vi "CharEditor.vi"() -> ()   [LabVIEW 2018]
uses:
  TypDefs/Char_Enum.ctl
panel:
  in  "ReplaceColor":bool
  in  "Color 2":u8(ring)=2
  in  "Color 1":u8(ring)
  out "Blue_LUT":bool[](array[boolean])
  out "Green_LUT":bool[](array[boolean])
  out "Red_LUT":bool[](array[boolean])
  in  "Create LUT":bool
  in  "Fill Column":bool
  in  "Color":u8(ring)
  in  "Fill Row":bool
  in  "Column":i32 min=0 max=24 step=1
  in  "Row":i32 min=0 max=24 step=1
  in  "Clear tile":bool
  in  "Rotate tile":bool
  in  "Paste tile":bool
  in  "Copy tile":bool
  in  "Save Tileset":bool
  in  "Active char":T1
  in  "25x25 Tile":u8[][](array[ring])
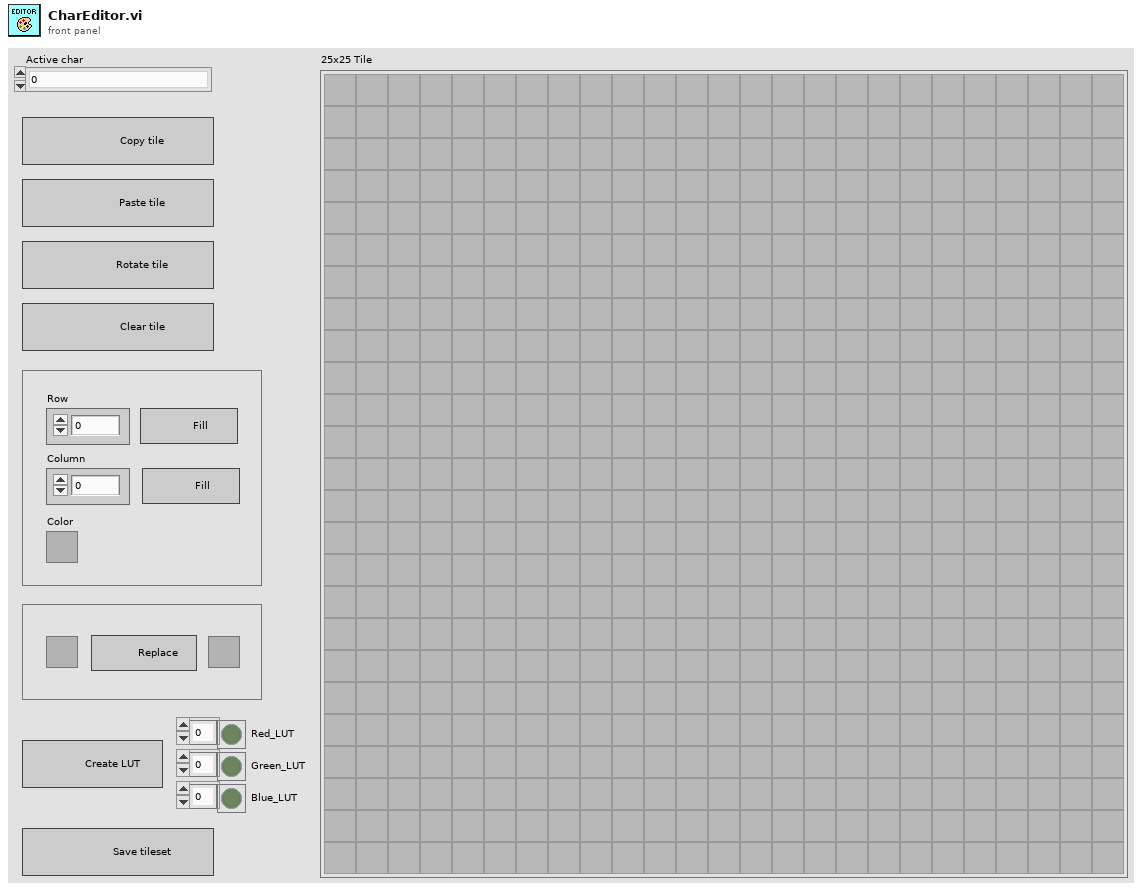
[diagram p1: front panel]
types:
  T1 = typedef "Char_Enum.ctl" = enum8{"0", "1", "2", "3", "4", "5", "6", "7", "8", "9"}
  T2 = cluster{"FilePath":path, "ActiveChar":T1, "TileSizeX":i32, "TileSizeY":i32, "Tileset":u8[][][], "Copy":u8[][]}
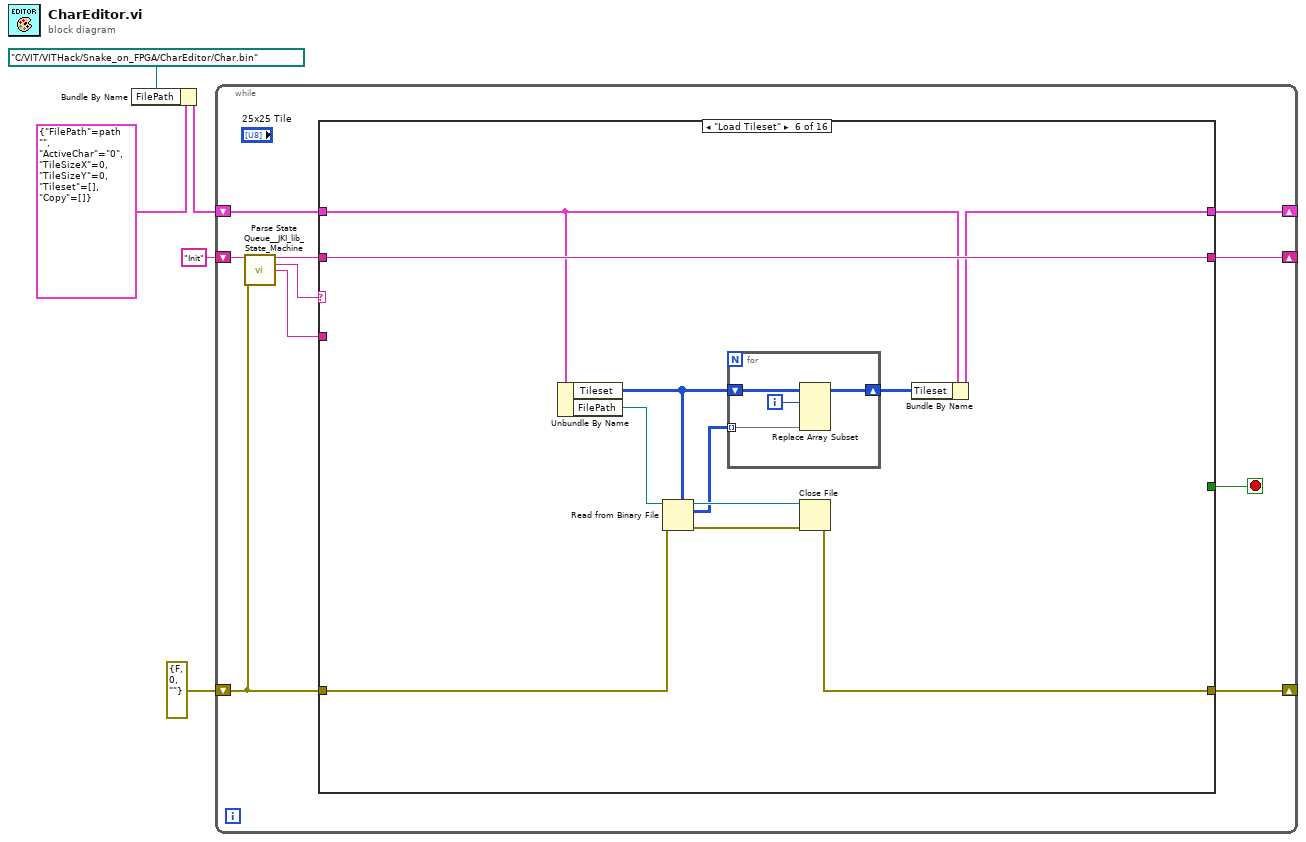
[diagram p0: block diagram]
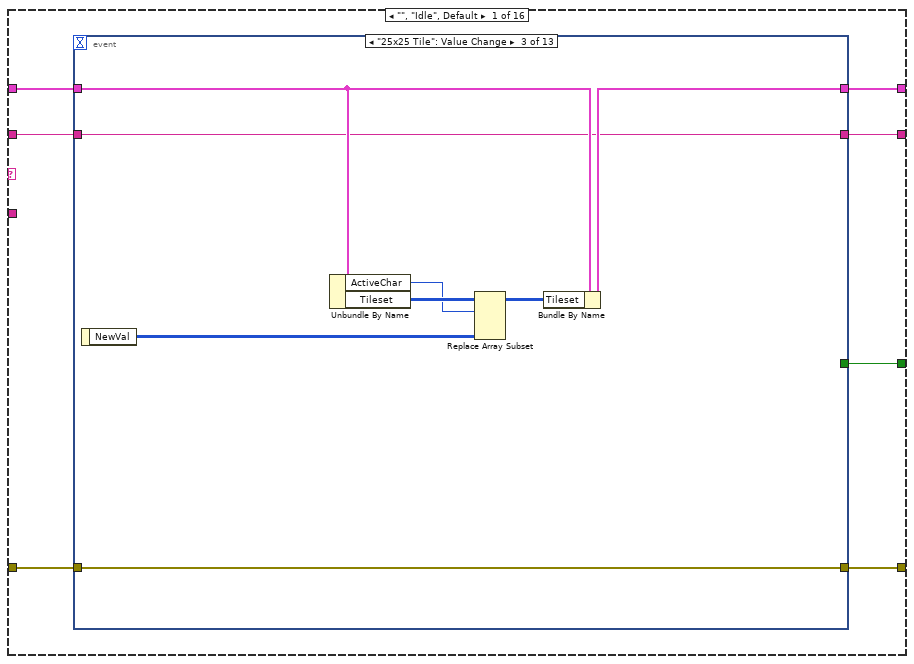
[diagram p2: hidden frame]
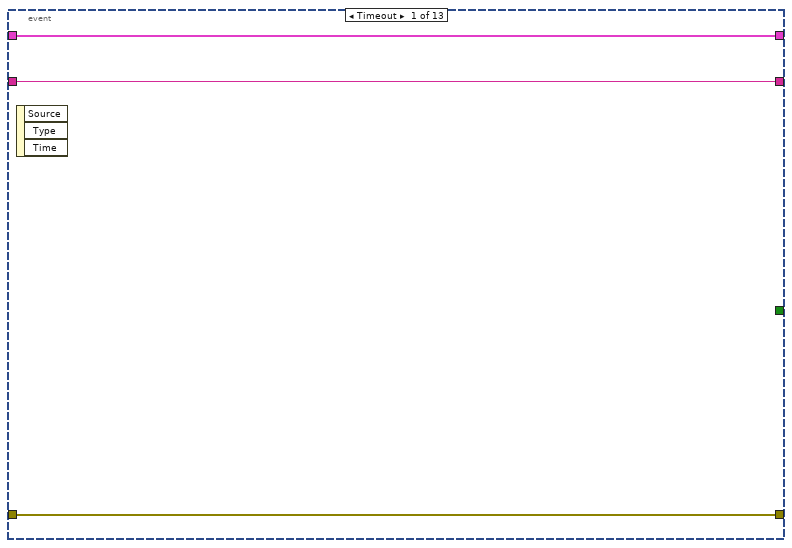
[diagram p3: hidden frame]
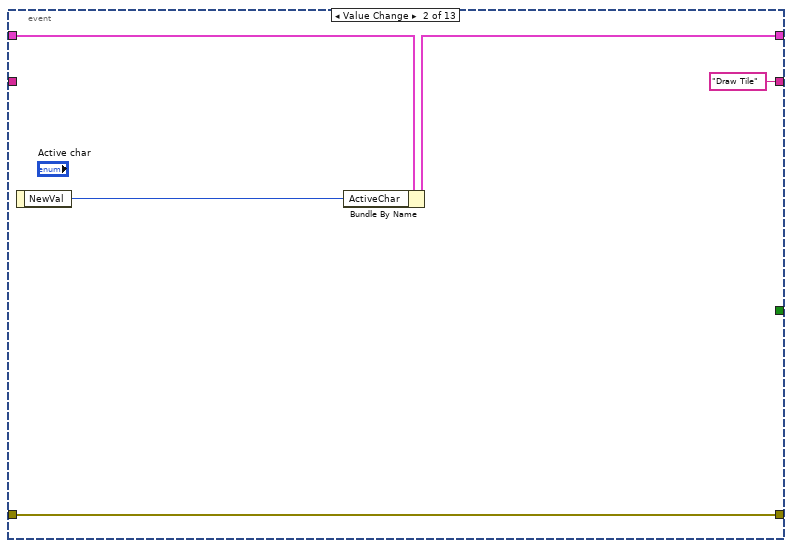
[diagram p4: hidden frame]
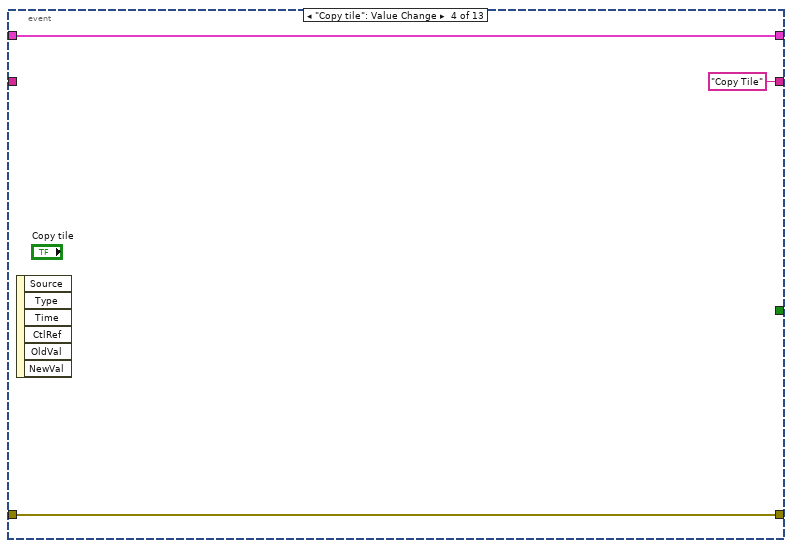
[diagram p5: hidden frame]
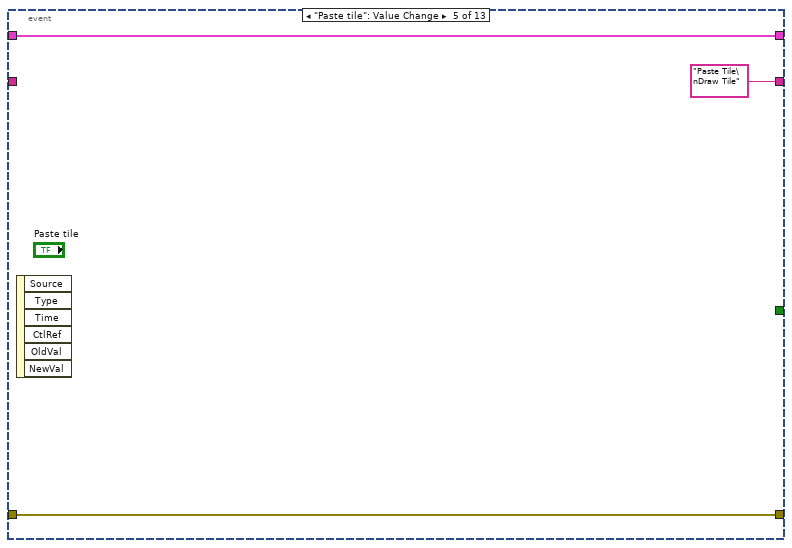
[diagram p6: hidden frame]
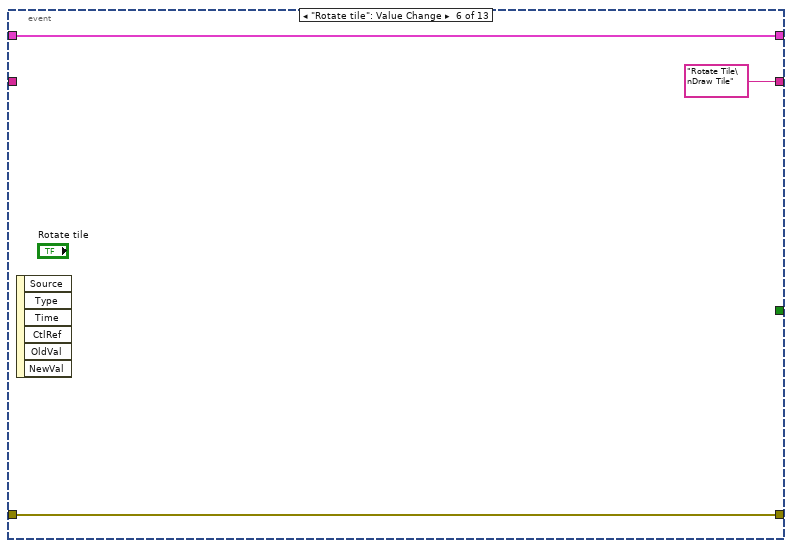
[diagram p7: hidden frame]
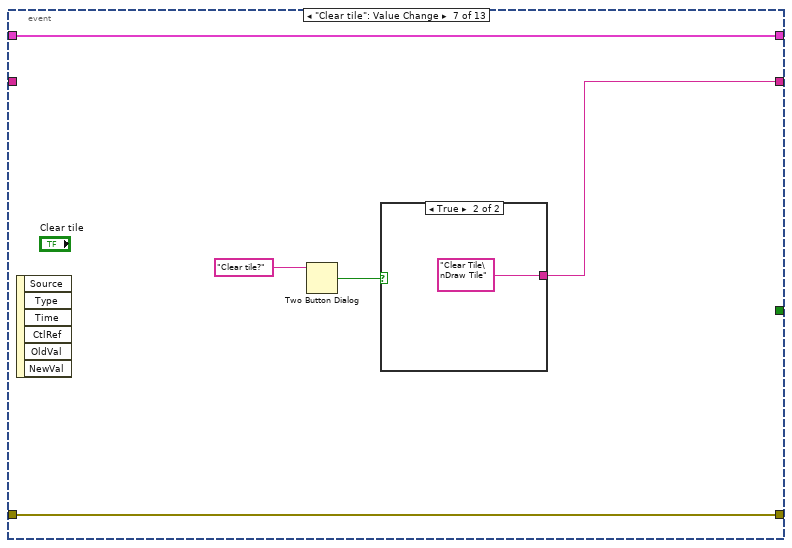
[diagram p8: hidden frame]
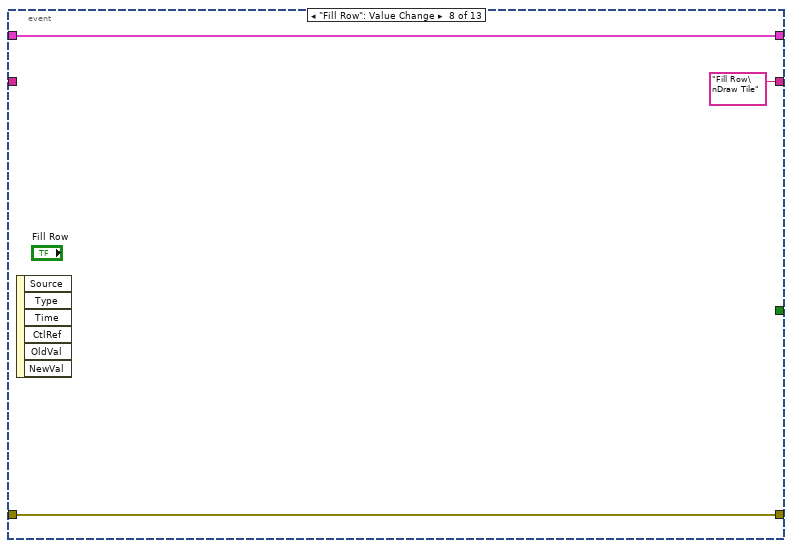
[diagram p10: hidden frame]
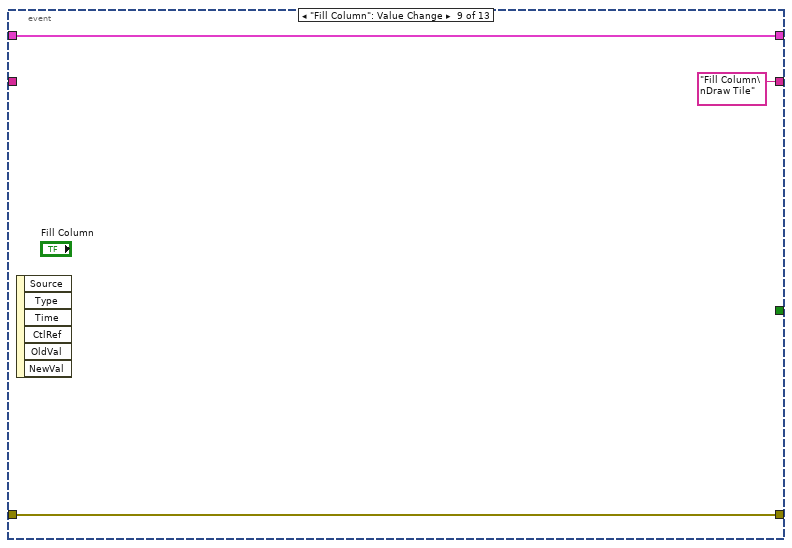
[diagram p11: hidden frame]
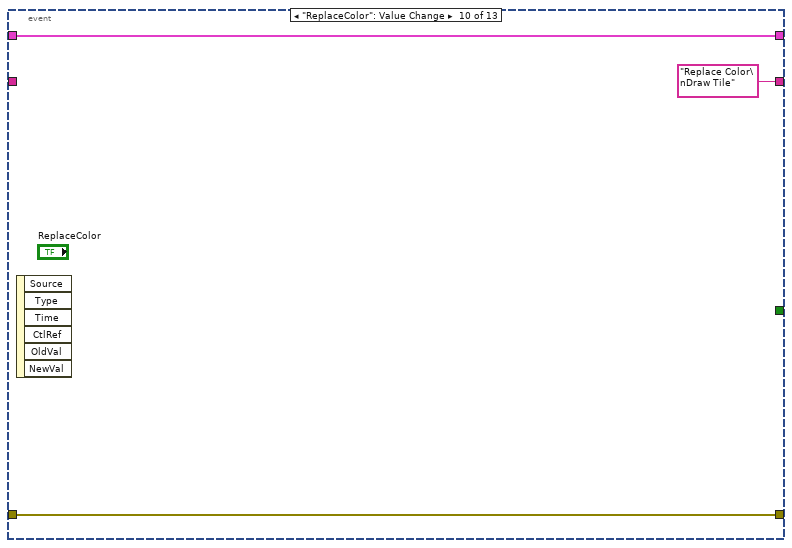
[diagram p12: hidden frame]
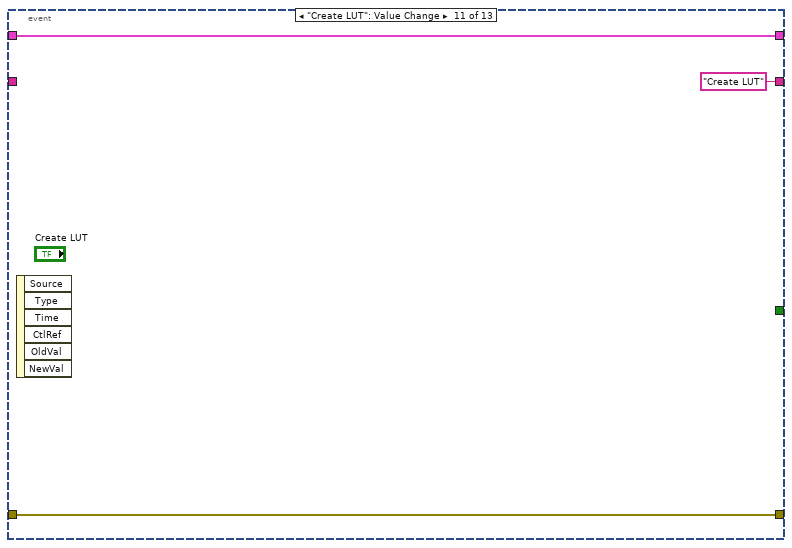
[diagram p13: hidden frame]
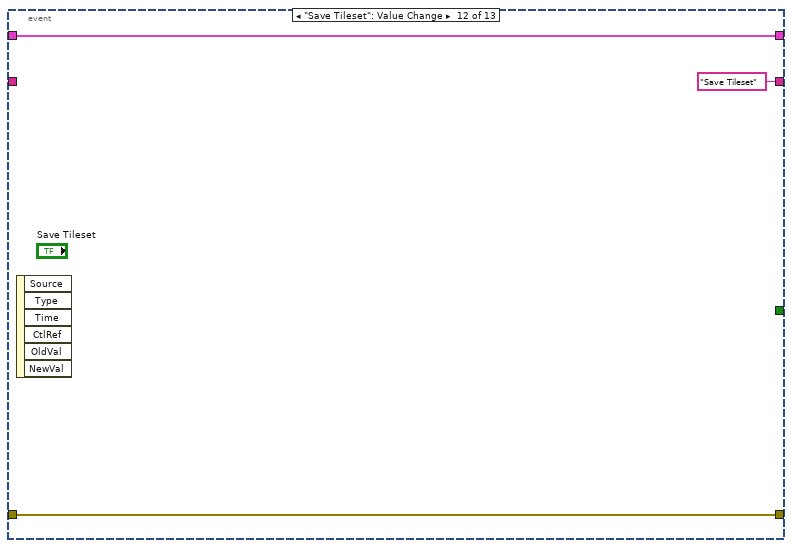
[diagram p14: hidden frame]
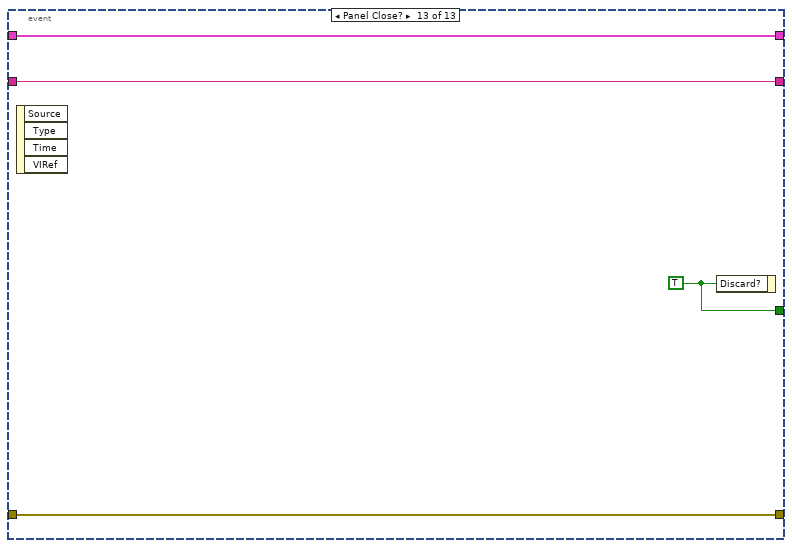
[diagram p15: hidden frame]
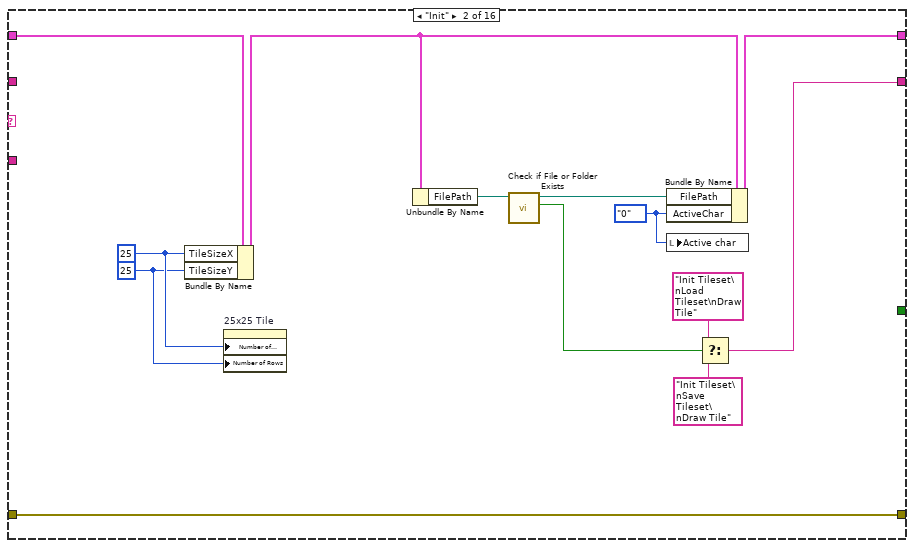
[diagram p16: hidden frame]
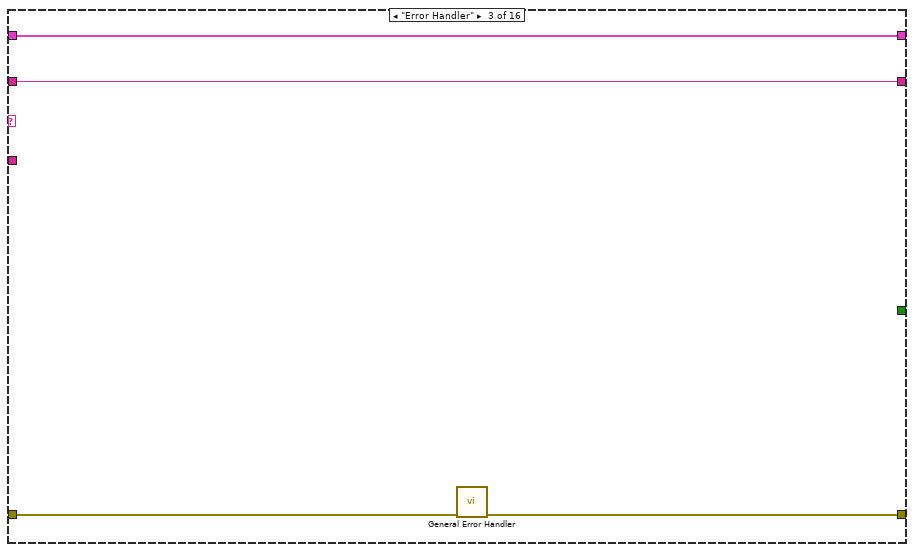
[diagram p17: hidden frame]
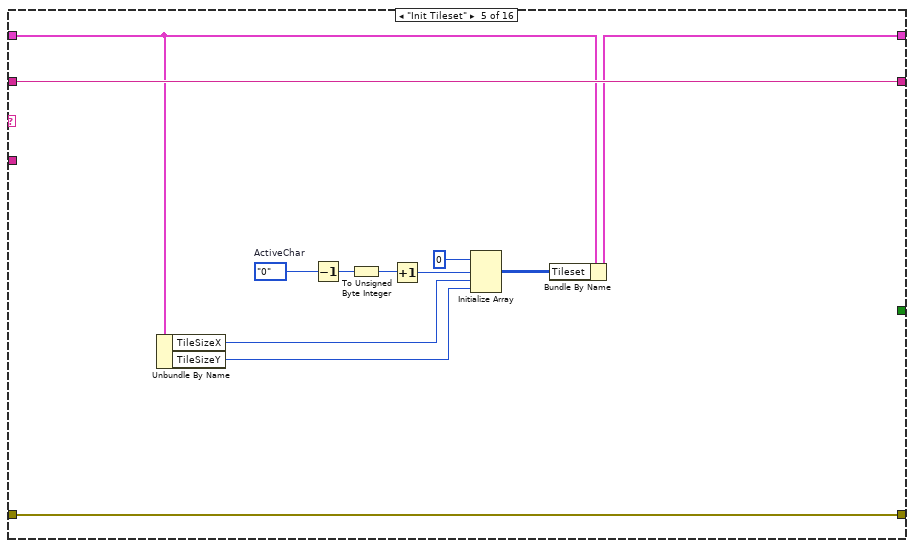
[diagram p19: hidden frame]
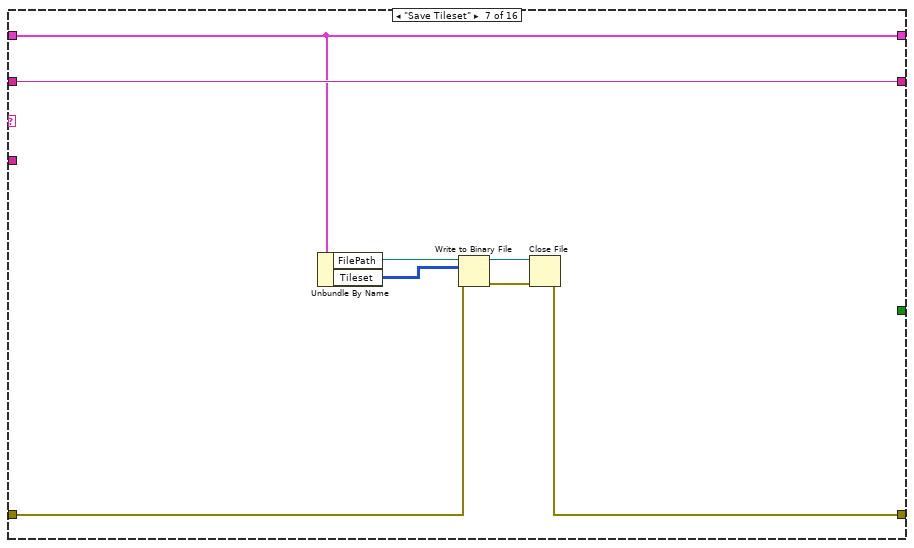
[diagram p20: hidden frame]
diagram:
  n1 = Bundle By Name(cluster=T2 {"FilePath"=path "", "ActiveChar"=enum."0", "TileSizeX"=0, "TileSizeY"=0, "Tileset"=[], "Copy"=[]}, "FilePath"=path "C:/VIT/VITHack/Snake_on_FPGA/CharEditor/Char.bin") -> (w2:T2)
  n2 = while {
    shift-right: [w14] -> _
    shift-left: "Init" ("Remaining States") -> [w15]
    shift-right: [w11] -> _
    shift-left: errorcluster {"status"=FALSE, "code"=0, "source"=""} ("error constant") -> [w10]
    shift-right: [w7] -> _
    shift-left: w2 -> [w8]
    stop <- w6 stop-if-true
    n3 = call <vilib>:"Parse State Queue__JKI_lib_State_Machine.vi"("State Queue"=w15, "Error In (no error)"=w10) -> ("Remaining States"=w13:string, "Current State"=w12:string, "Arguments"=w9:string)  [unwired: 11 in]
    n4 = case shown="\"Load Tileset\"" w12 {
      tunnel: [w22 w79 w89 w92 w104 w115 w127 w134 w141 w142 w156 w169 w180 w191 w200 w220] -> w14
      tunnel: w13 -> [w21 _ w89 w92 w104 w115 w127 w134 w141 w142 w156 w169 w180 w191 w200 w220]
      tunnel: [w20 w85 w87 w91 w103 w109 w120 w129 w140 w149 w159 w172 w183 w194 w203 w219] -> w11
      tunnel: w10 -> [w19 w85 w88 w91 w103 w112 w123 w128 w140 w149 w159 w172 w183 w194 w203 w219]
      tunnel: w9 -> [_ _ _ _ _ _ _ _ _ _ _ _ _ _ _ _]
      tunnel: w8 -> [w18 w84 w86 w90 w95 w114 w126 w133 w139 w148 w158 w171 w182 w193 w202 w218]
      tunnel: [w17 w83 w86 w90 w97 w108 w126 w133 w136 w145 w157 w170 w181 w192 w201 w218] -> w7
      tunnel: [w16 _ _ _ _ _ _ _ _ _ _ _ _ _ _ _] -> w6
      frame "", "Idle", Default {
        n5 = event shown="[2] \"25x25 Tile\": Value Change" {
          selector: _ -> [_ _ _ _ _ _ _ _ _ _ _ _ _]
          dyn-events: _ -> [_ _ _ _ _ _ _ _ _ _ _ _ _]
          timeout: _ -> [_ _ _ _ _ _ _ _ _ _ _ _ _]
          tunnel: [w25 "Draw Tile" ("Remaining States") w31 "Copy Tile" ("Remaining States") "Paste Tile\nDraw Tile" ("Remaining States") "Rotate Tile\nDraw Tile" ("Remaining States") w50 "Fill Row\nDraw Tile" ("Remaining States") "Fill Column\nDraw Tile" ("Remaining States") "Replace Color\nDraw Tile" ("Remaining States") "Create LUT" ("Remaining States") "Save Tileset" ("Remaining States") w72] -> w22
          tunnel: w21 -> [w25 _ w31 _ _ _ _ _ _ _ _ _ w72]
          tunnel: [w24 w30 w38 w41 w44 w47 w52 w56 w59 w62 w65 w68 w71] -> w20
          tunnel: w19 -> [w24 w30 w38 w41 w44 w47 w52 w56 w59 w62 w65 w68 w71]
          tunnel: w18 -> [w23 w29 w36 w40 w43 w46 w51 w55 w58 w61 w64 w67 w70]
          tunnel: [w23 w28 w37 w40 w43 w46 w51 w55 w58 w61 w64 w67 w70] -> w17
          tunnel: [_ _ _ _ _ _ _ _ _ _ _ _ w69] -> w16
          event Timeout {
            n6 = event-data() -> ()  [unwired: 1 in, 3 out]
          }
          event Value Change {
            n7 = event-data() -> ("NewVal"=w27:T1)  [unwired: 1 in]
            n8 = Bundle By Name(cluster=w29, "ActiveChar"=w27) -> (w28:T2)
          }
          event "25x25 Tile": Value Change {
            n9 = event-data() -> ("NewVal"=w33:u8[][])  [unwired: 1 in]
            n10 = Unbundle By Name(w36) -> ("ActiveChar"=w32:T1, "Tileset"=w35:u8[][][])
            n11 = Replace Array Subset(array=w35, new element=w33, index (dim 0)=w32) -> (w34:u8[][][])  [unwired: 2 in]
            n12 = Bundle By Name(cluster=w36, "Tileset"=w34) -> (w37:T2)
          }
          event "Copy tile": Value Change {
            n13 = event-data() -> ()  [unwired: 1 in, 6 out]
          }
          event "Paste tile": Value Change {
            n14 = event-data() -> ()  [unwired: 1 in, 6 out]
          }
          event "Rotate tile": Value Change {
            n15 = event-data() -> ()  [unwired: 1 in, 6 out]
          }
          event "Clear tile": Value Change {
            n16 = event-data() -> ()  [unwired: 1 in, 6 out]
            n17 = Two Button Dialog(message="Clear tile?") -> (T button?=w48:bool)  [unwired: 2 in]
            n18 = case shown="True" w48 {
              tunnel: [_ "Clear Tile\nDraw Tile" ("Remaining States")] -> w50
              frame False {
              }
              frame True {
              }
            }
          }
          event "Fill Row": Value Change {
            n19 = event-data() -> ()  [unwired: 1 in, 6 out]
          }
          event "Fill Column": Value Change {
            n20 = event-data() -> ()  [unwired: 1 in, 6 out]
          }
          event "ReplaceColor": Value Change {
            n21 = event-data() -> ()  [unwired: 1 in, 6 out]
          }
          event "Create LUT": Value Change {
            n22 = event-data() -> ()  [unwired: 1 in, 6 out]
          }
          event "Save Tileset": Value Change {
            n23 = event-data() -> ()  [unwired: 1 in, 6 out]
          }
          event Panel Close? {
            w69 = TRUE ("Discard?")
            n24 = event-data() -> ()  [unwired: 1 in, 4 out]
            n25 = event-data("Discard?"=w69) -> ()  [unwired: 1 in, 1 out]
          }
        }
      }
      frame "Init" {
        w75 = 25 ("TileSizeY")
        w76 = 25 ("TileSizeX")
        w77 = Char_Enum."0" ("ActiveTile")
        n26 = Bundle By Name(cluster=w84, "TileSizeX"=w76, "TileSizeY"=w75) -> (w74:T2)
        n27 = property on="25x25 Tile" class="Arr (strict)"("Number of Columns"=w76, "Number of Rows"=w75) -> ()  [unwired: 2 in, 2 out]
        n28 = Unbundle By Name(w74) -> ("FilePath"=w73:path)
        n29 = call <vilib>:"Check if File or Folder Exists.vi"("path"=w73) -> ("file or folder exists?"=w78:bool, "dup path"=w82:path)  [unwired: 8 in, 1 out]
        n30 = Bundle By Name(cluster=w74, "FilePath"=w82, "ActiveChar"=w77) -> (w83:T2)
        n31 = local write "Active char"(w77) -> ()
        n32 = Select(t="Init Tileset\nLoad Tileset\nDraw Tile", s=w78, f="Init Tileset\nSave Tileset\nDraw Tile") -> (s? t:f=w79:string)
      }
      frame "Error Handler" {
        n33 = call <vilib>:"General Error Handler.vi"("error in (no error)"=w88) -> ("error out"=w87:errorcluster)  [unwired: 10 in, 4 out]
      }
      frame "------ Functions ------" {
      }
      frame "Init Tileset" {
        w102 = Char_Enum."0"  # ActiveChar
        n34 = Unbundle By Name(w95) -> ("TileSizeX"=w94:i32, "TileSizeY"=w93:i32)
        n35 = Decrement(x=w102) -> (x-1=w101:T1)
        n36 = To Unsigned Byte Integer(number=w101) -> (unsigned 8bit integer=w100:u8)
        n37 = Increment(x=w100) -> (x+1=w99:u8)
        n38 = Initialize Array(u8 0, w99, w94, w93) -> (w96:u8[][][])
        n39 = Bundle By Name(cluster=w95, "Tileset"=w96) -> (w97:T2)
      }
      frame "Load Tileset" {
        n40 = Unbundle By Name(w114) -> ("Tileset"=w107:u8[][][], "FilePath"=w113:path)
        n41 = Read from Binary File(5:w107, 8:w112, 11:w113) -> (0:w110:errorcluster, 2:w106:u8[][][], 3:w111:refnum<file>)  [unwired: 3 in, 1 out]
        n42 = for {
          tunnel: w106 -> [w118] mode=indexing
          shift-right: [w117] -> w105
          shift-left: w107 -> [w119]
          i -> [w116]
          n43 = Replace Array Subset(array=w119, new element=w118, index (dim 0)=w116) -> (w117:u8[][][])  [unwired: 2 in]
        }
        n44 = Close File(refnum=w111, error in=w110) -> (error out=w109:errorcluster)  [unwired: 1 out]
        n45 = Bundle By Name(cluster=w114, "Tileset"=w105) -> (w108:T2)
      }
      frame "Save Tileset" {
        n46 = Unbundle By Name(w126) -> ("FilePath"=w125:path, "Tileset"=w124:u8[][][])
        n47 = Write to Binary File(file (use dialog)=w125, data=w124, error in=w123) -> (refnum out=w122:refnum<file>, error out=w121:errorcluster)  [unwired: 3 in, 1 out]
        n48 = Close File(refnum=w122, error in=w121) -> (error out=w120:errorcluster)  [unwired: 1 out]
      }
      frame "Draw Tile" {
        n49 = Unbundle By Name(w133) -> ("Tileset"=w132:u8[][][], "ActiveChar"=w131:T1)
        n50 = Index Array(array=w132, index (dim 0)=w131) -> (element=w130:u8[][])  [unwired: 2 in]
        n51 = property on="25x25 Tile" class="Arr (strict)"(error in=w128, "Value"=w130) -> (error out=w129:errorcluster)  [unwired: 1 in, 1 out]
      }
      frame "Copy Tile" {
        n52 = Unbundle By Name(w139) -> ("Tileset"=w138:u8[][][], "ActiveChar"=w137:T1)
        n53 = Index Array(array=w138, index (dim 0)=w137) -> (element=w135:u8[][])  [unwired: 2 in]
        n54 = Bundle By Name(cluster=w139, "Copy"=w135) -> (w136:T2)
      }
      frame "Paste Tile" {
        n55 = Unbundle By Name(w148) -> ("Tileset"=w147:u8[][][], "ActiveChar"=w146:T1, "Copy"=w143:u8[][])
        n56 = Replace Array Subset(array=w147, new element=w143, index (dim 0)=w146) -> (w144:u8[][][])  [unwired: 2 in]
        n57 = Bundle By Name(cluster=w148, "Tileset"=w144) -> (w145:T2)
      }
      frame "Rotate Tile" {
        n58 = Unbundle By Name(w158) -> ("Tileset"=w154:u8[][][], "ActiveChar"=w152:T1)
        n59 = Index Array(array=w154, index (dim 0)=w152) -> (element=w155:u8[][])  [unwired: 2 in]
        n60 = Transpose 2D Array(2D array=w155) -> (transposed array=w151:u8[][])
        n61 = for {
          tunnel: w151 -> [w161] mode=indexing
          tunnel: [w160] -> w150 mode=indexing
          n62 = Reverse 1D Array(array=w161) -> (reversed array=w160:u8[])
        }
        n63 = Replace Array Subset(array=w154, new element=w150, index (dim 0)=w152) -> (w153:u8[][][])  [unwired: 2 in]
        n64 = Bundle By Name(cluster=w158, "Tileset"=w153) -> (w157:T2)
      }
      frame "Clear Tile" {
        n65 = Unbundle By Name(w171) -> ("Tileset"=w168:u8[][][], "ActiveChar"=w166:T1, "TileSizeX"=w165:i32, "TileSizeY"=w164:i32)
        n66 = Initialize Array(u8 0 ("element"), w165, w164) -> (w162:u8[][])
        n67 = Replace Array Subset(array=w168, new element=w162, index (dim 0)=w166) -> (w167:u8[][][])  [unwired: 2 in]
        n68 = Bundle By Name(cluster=w171, "Tileset"=w167) -> (w170:T2)
      }
      frame "Fill Row" {
        n69 = Unbundle By Name(w182) -> ("Tileset"=w179:u8[][][], "ActiveChar"=w177:T1, "TileSizeY"=w175:i32)
        n70 = local read "Color"() -> (w176:u8)
        n71 = Initialize Array(w176, w175) -> (w174:u8[])
        n72 = Replace Array Subset(array=w179, new element=w174, index (dim 0)=w177, index (dim 1)="Row") -> (w178:u8[][][])  [unwired: 1 in]
        n73 = Bundle By Name(cluster=w182, "Tileset"=w178) -> (w181:T2)
      }
      frame "Fill Column" {
        n74 = Unbundle By Name(w193) -> ("Tileset"=w190:u8[][][], "ActiveChar"=w188:T1, "TileSizeX"=w187:i32)
        n75 = Initialize Array("Color", w187) -> (w186:u8[])
        n76 = Replace Array Subset(array=w190, new element=w186, index (dim 0)=w188, index (dim 2)="Column") -> (w189:u8[][][])  [unwired: 1 in]
        n77 = Bundle By Name(cluster=w193, "Tileset"=w189) -> (w192:T2)
      }
      frame "Replace Color" {
        n78 = Unbundle By Name(w202) -> ("Tileset"=w198:u8[][][], "ActiveChar"=w197:T1)
        n79 = Index Array(array=w198, index (dim 0)=w197) -> (element=w199:u8[][])  [unwired: 2 in]
        n80 = for {
          tunnel: w199 -> [w205] mode=indexing
          tunnel: [w204] -> w196 mode=indexing
          n81 = for {
            tunnel: w205 -> [w207] mode=indexing
            tunnel: [w206] -> w204 mode=indexing
            n82 = Equal?(x=w207, y="Color 1") -> (x = y?=w209:bool)
            n83 = Select(t="Color 2", s=w209, f=w207) -> (s? t:f=w206:u8)
          }
        }
        n84 = Replace Array Subset(array=w198, new element=w196, index (dim 0)=w197) -> (w195:u8[][][])  [unwired: 2 in]
        n85 = Bundle By Name(cluster=w202, "Tileset"=w195) -> (w201:T2)
      }
      frame "Create LUT" {
        n86 = Unbundle By Name(w218) -> ("Tileset"=w217:u8[][][], "TileSizeX"=w216:i32, "TileSizeY"=w215:i32)
        n87 = Multiply(x=w216, y=w215) -> (x*y=w214:i32)
        n88 = for "Iterate trough tiles" {
          tunnel: w217 -> [w226] mode=indexing
          tunnel: w214 -> [w225]
          tunnel: [w223] -> w213 mode=concatenating
          tunnel: [w222] -> w212 mode=concatenating
          tunnel: [w221] -> w211 mode=concatenating
          n89 = Reshape Array(w226, w225) -> (w224:u8[])
          n90 = for "Iterate trough pixels" {
            tunnel: w224 -> [w230] mode=indexing
            tunnel: [w229] -> w223 mode=indexing
            tunnel: [w228] -> w222 mode=indexing
            tunnel: [w227] -> w221 mode=indexing
            n91 = case shown="0, Default" w230 {
              tunnel: [w233 w236 w239 w242 w245 w248 w251 w254] -> w229
              tunnel: [w232 w235 w238 w241 w244 w247 w250 w253] -> w228
              tunnel: [w231 w234 w237 w240 w243 w246 w249 w252] -> w227
              frame 0, Default {
                w231 = FALSE  # B
                w232 = FALSE  # G
                w233 = FALSE  # R
                # "Black"
              }
              frame 1 {
                w234 = FALSE  # B
                w235 = FALSE  # G
                w236 = TRUE  # R
                # "Red"
              }
              frame 2 {
                w237 = FALSE  # B
                w238 = TRUE  # G
                w239 = FALSE  # R
                # "Green"
              }
              frame 3 {
                w240 = TRUE  # B
                w241 = FALSE  # G
                w242 = FALSE  # R
                # "Blue"
              }
              frame 4 {
                w243 = TRUE  # B
                w244 = TRUE  # G
                w245 = FALSE  # R
                # "Cyan"
              }
              frame 5 {
                w246 = TRUE  # B
                w247 = FALSE  # G
                w248 = TRUE  # R
                # "Purple"
              }
              frame 6 {
                w249 = FALSE  # B
                w250 = TRUE  # G
                w251 = TRUE  # R
                # "Yellow"
              }
              frame 7 {
                w252 = TRUE  # B
                w253 = TRUE  # G
                w254 = TRUE  # R
                # "White"
              }
            }
          }
        }
        "Red_LUT" <- w213
        "Green_LUT" <- w212
        "Blue_LUT" <- w211
      }
    }
  }
